vi "FTW-Messenger-Actor-CheckShutdown.vi"(0 "Messenger":refnum<class "FTW-Messenger-Actor.lvclass">, 11 "error in":errorcluster) -> (4 "Messenger out":refnum<class "FTW-Messenger-Actor.lvclass">, 6 "Shutdown Payload Message":refnum<class "FTW-Message.lvclass">, 8 "Shutdown Requested":bool, 15 "error out":errorcluster)   [LabVIEW 2012, in "FTW-Messenger-Actor.lvclass"]
uses:
  FTW-Messenger-Actor.lvclass
  Message/FTW-Message.lvclass
  FTW-Messenger-Actor.lvclass/FTW-Messenger-Actor.ctl
panel:
  # "Inputs"
  # "Outputs"
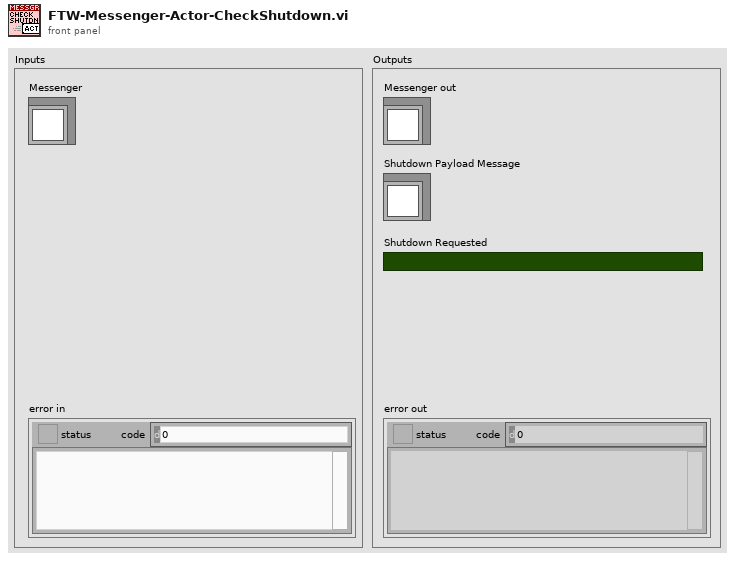
[diagram p1: front panel]
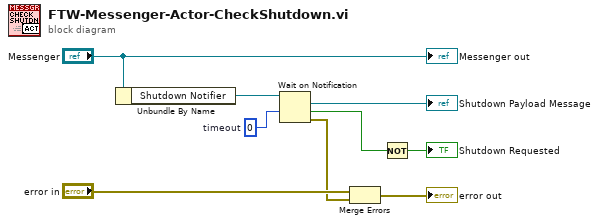
[diagram p0: block diagram]
diagram:
  w5 = 0  # timeout
  n1 = Unbundle By Name("Messenger") -> ("Shutdown Notifier"=w6:refnum<notifier>)
  n2 = Wait on Notification(notifier=w6, timeout in ms (-1)=w5) -> (notification=→"Shutdown Payload Message":refnum<class "FTW-Message.lvclass">, timed out?=w4:bool, error out=w2:errorcluster)  [unwired: 2 in, 1 out]
  n3 = Merge Errors("error in", w2) -> (→"error out":errorcluster)
  n4 = Not(x=w4) -> (.not. x?=→"Shutdown Requested":bool)
  "Messenger out" <- "Messenger"
